vi "Error Logging.vi"() -> ()   [LabVIEW 2014]
panel:
  out "queue out":refnum<queue>
  in  "queue in":refnum<queue>
  out "error out":errorcluster
  in  "error in (no error)":errorcluster
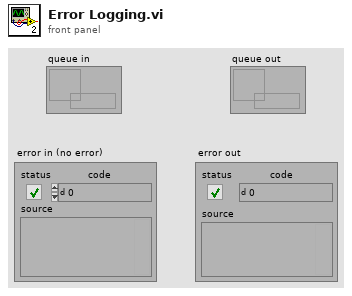
[diagram p1: front panel]
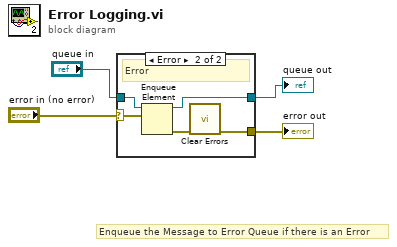
[diagram p0: block diagram]
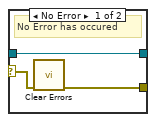
[diagram p2: hidden frame]
diagram:
  # "Enqueue the Message to Error Queue if there is an Error"
  n1 = case shown="Error" "error in (no error)" {
    selector: "error in (no error)" -> [w7 w10]
    tunnel: "queue in" -> [w5 w12]
    tunnel: [w5 w11] -> w3
    tunnel: [w6 w8] -> w1
    frame No Error {
      # "No Error has occured"
      n2 = call <vilib>:"Clear Errors.vi"("error in (no error)"=w7) -> ("error out"=w6:errorcluster)  [unwired: 5 in, 1 out]
    }
    frame Error {
      # "Error"
      n3 = Enqueue Element(queue=w12, element=w10) -> (queue out=w11:refnum<queue>, error out=w9:errorcluster)  [unwired: 2 in, 1 out]
      n4 = call <vilib>:"Clear Errors.vi"("error in (no error)"=w9) -> ("error out"=w8:errorcluster)  [unwired: 5 in, 1 out]
    }
  }
  "error out" <- w1
  "queue out" <- w3
